vi "Create DataTable.vi"(8 "错误输入（无错误）":errorcluster, 11 "tableName":string) -> (0 "错误输出":errorcluster, 3 "DataTable":refnum<k24>)   [LabVIEW 2012, in "DataGridView.lvlib"]
uses:
  DataGridView.lvlib
  System.Data
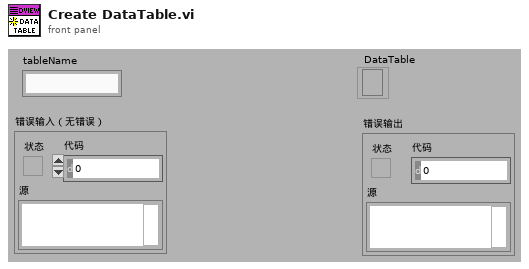
[diagram p1: front panel]
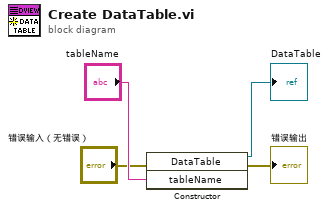
[diagram p0: block diagram]
diagram:
  n1 = constructor class="DataTable"(error in="错误输入（无错误）", "tableName"="tableName") -> (reference out=→"DataTable":refnum<k24>, error out=→"错误输出":errorcluster)  [unwired: 2 in, 2 out]
